vi "Stop Core.vi"(10 "final error code":i32, 11 "TDMS File Writer in":refnum<class "File Writer_TDMS.lvclass">) -> (3 "TDMS File Writer out":refnum<class "File Writer_TDMS.lvclass">)   [LabVIEW 2020, in "File Writer_TDMS.lvlib" / "File Writer_TDMS.lvclass"]
doc: "(<B>Filename</B>: Actor Framework.lvlib:Actor.lvclass:Stop Core.vi)\n\nDefines what the actor does before it stops. Use the <B>final error code</B> input to determine whether the actor shut down in response to an error.\n\nThis implementation closes the TDMS file if the file was active."
uses:
  File Writer_TDMS.lvclass
  PPL/HDH.Actor Framework.Core.File Writer.lvlibp/File Writer/File Writer.lvclass
  C:/Current projects/WS/PPL/HDH.Actor Framework.Core.File Writer.lvlibp/File Writer/File Writer.lvclass
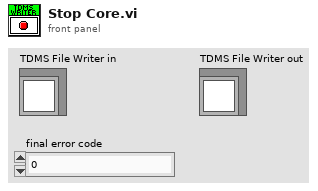
[diagram p1: front panel]
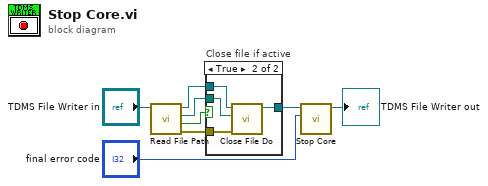
[diagram p0: block diagram]
diagram:
  n1 = call "Read File Path.vi"("File Writer in"="TDMS File Writer in") -> ("error out"=w1:errorcluster, "Is Active?"=w5:bool, "File Path"=w2:path, "File Writer out"=w4:refnum<class "File Writer_TDMS.lvclass">)  [unwired: 7 in]
  n2 = case "Close file if active" shown="True" w5 {
    tunnel: w4 -> [w9 w13]
    tunnel: [w9 w12] -> w3
    tunnel: w2 -> [_ w11]
    tunnel: w1 -> [_ w10]
    frame False {
    }
    frame True {
      n3 = call-dynamic "Close File Do.vi"("error in (no error)"=w10, "File Path"=w11, "TDMS File Writer in"=w13) -> ("TDMS File Writer out"=w12:refnum<class "File Writer_TDMS.lvclass">)  [unwired: 7 in, 1 out]
    }
  }
  n4 = call-parent "Stop Core.vi"("final error code"="final error code", "Actor in"=w3) -> ("Actor out"=→"TDMS File Writer out":refnum<class "File Writer_TDMS.lvclass">)  [unwired: 9 in]
